vi "3458A Digitizing Process.vi"(8 "error in":errorcluster, 11 "session in":variant) -> (0 "error out":errorcluster, 3 "aux data out":variant)   [LabVIEW 2018, in "3458A Virtual Digitizer.lvlib"]
doc: "3458A digitizing lib: Main digitizing process. The VI is assynchronously executed once for each channel (all in parallel). It is started by calling 'Initiate Digitizing Process'. It then samples and sends the digitized data via queues to main process where the data are collected using 'Fetch Digitized Data'. Configuration of the execution is stored in 'session in' variable, execution control details are in 'session in->proc setup' cluster. Each instance of this VI has ID starting from 0 which identifies to which channel it belongs to."
uses:
  3458A Virtual Digitizer.lvlib
  3458A Digitizer Session.ctl
  3458A Virtual Channel Config.ctl
  Counter/Counter Session.ctl
  Counter/Counter Type.ctl
  AWG/AWG Session.ctl
  AWG/AWG Type.ctl
  3458A Sync Mode.ctl
  3458A Idn Mode.ctl
  3458A Digitizing Low Levels/Configure/Sampling Mode.ctl
  3458A Digitizing Process Options.ctl
  3458A Data Packet.ctl
  3458A Aux Record Data.ctl
  3458A Digitizing Low Levels/Configure/Level Setup.ctl
  3458A Digitizing Low Levels/Configure/First Sample Trigger.ctl
  3458A Aperture Selection Mode.ctl
  <vilib>/Utility/error.llb/Error Cluster From Error Code.vi
  <vilib>/ErrorRing/Error Ring.xnode
  Counter/Counter.lvlib
  AWG/AWG.lvlib
  3458A Digitizing Low Levels/3458A Digitizing Low Levels.lvlib
  3458A Basic Driver/3458A Basic Driver.lvlib
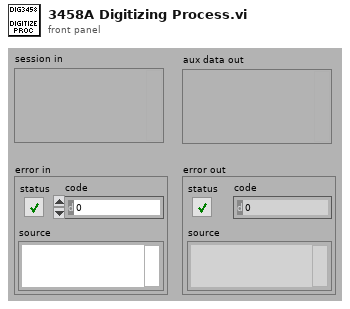
[diagram p1: front panel]
types:
  T1 = typedef "3458A Virtual Digitizer.lvlib/3458A Digitizing Low Levels.lvlib/First Sample Trigger.ctl" = enum16{"AUTO", "EXT", "SYN", "SGL", "HOLD", "LEVEL"}
  T2 = typedef "3458A Virtual Digitizer.lvlib/3458A Data Packet.ctl" = cluster{"data":i32[][], "offset [smpl]":i32, "count [smpl]":i32, "all done?":bool, "sampling?":bool, "queue buffer [%]":dbl, "valid?":bool}
  T3 = typedef "3458A Virtual Digitizer.lvlib/3458A Digitizer Session.ctl" = cluster{"channels":T4[], "sync unit":T5, "awg unit":T7, "sync mode":T9, "streaming mode":bool, "idn mode":T10, "sampling mode":T11, "Ts [s]":dbl, "sample memory [B]":i32, "proc setup":T12, "sample size [B]":i32, "sample count":i32, "aux data":T14, "ranges [V]":dbl[], "aperture [s]":dbl, "LEVEL trigger":T15, "trigger mode":T1, "measure temp.?":bool, "disp mesages":string[], "shared bus?":bool, "disable display?":bool, "aper mode":T16, "aper rules":dbl[][]}
  T4 = typedef "3458A Virtual Digitizer.lvlib/3458A Virtual Channel Config.ctl" = cluster{"VISA":refnum<visa-resource-name>, "Range [Vpk]":dbl, "btn clr":bool, "btn up":bool, "btn down":bool}
  T5 = typedef "Counter.lvlib/Counter Session.ctl" = cluster{"VISA":refnum<visa-resource-name>, "type":T6}
  T6 = typedef "Counter.lvlib/Counter Type.ctl" = enum16{"Picotest U6200A", "dummy"}
  T7 = typedef "AWG.lvlib/AWG Session.ctl" = cluster{"type":T8, "VISA":refnum<visa-resource-name>, "enable 10MHz ref":bool}
  T8 = typedef "AWG.lvlib/AWG Type.ctl" = enum16{"Agilent 331xxA to 332xxA", "Agilent 335xxA to 336xxA", "Tektronix AFG3101C", "dummy"}
  T9 = typedef "3458A Virtual Digitizer.lvlib/3458A Sync Mode.ctl" = enum16{"MASTER-SLAVE, MASTER clocked by TIMER", "MASTER-SLAVE, MASTER clocked by AWG", "ALL clocked by AWG", "MASTER-SLAVE, ALL clocked by TIMER", "ALL clocked by AWG with DFLL"}
  T10 = typedef "3458A Virtual Digitizer.lvlib/3458A Idn Mode.ctl" = enum16{"Auto", "Sequential (chn A, chn B, ...)", "From calibration string"}
  T11 = typedef "3458A Virtual Digitizer.lvlib/3458A Digitizing Low Levels.lvlib/Sampling Mode.ctl" = enum16{"DCV", "DSDC", "DSAC"}
  T12 = typedef "3458A Virtual Digitizer.lvlib/3458A Digitizing Process Options.ctl" = cluster{"channel id":i32, "packet size [smpl]":i32, "current timeout [s]":dbl, "blk2blk timeout [s]":dbl, "event time":timestamp, "stop notifier":refnum<notifier>, "data queues":refnum<queue>[], "proc refs":refnum<vi>[], "bus semaphore":T13}
  T13 = typedef "Semaphore RefNum" = refnum<k1>
  T14 = typedef "3458A Virtual Digitizer.lvlib/3458A Aux Record Data.ctl" = cluster{"channel id":i32, "valid?":bool[], "gain [V]":dbl[], "timestamp [s]":dbl[], "Ts [s]":dbl, "abs timestamp":timestamp, "t [deg C]":dbl[]}
  T15 = typedef "3458A Virtual Digitizer.lvlib/3458A Digitizing Low Levels.lvlib/Level Setup.ctl" = cluster{"edge":enum16{"POS", "NEG"}, "level [V]":dbl, "coupling":enum16{"DC", "AC"}}
  T16 = typedef "3458A Virtual Digitizer.lvlib/3458A Aperture Selection Mode.ctl" = enum16{"Manual", "Maximum", "Table"}
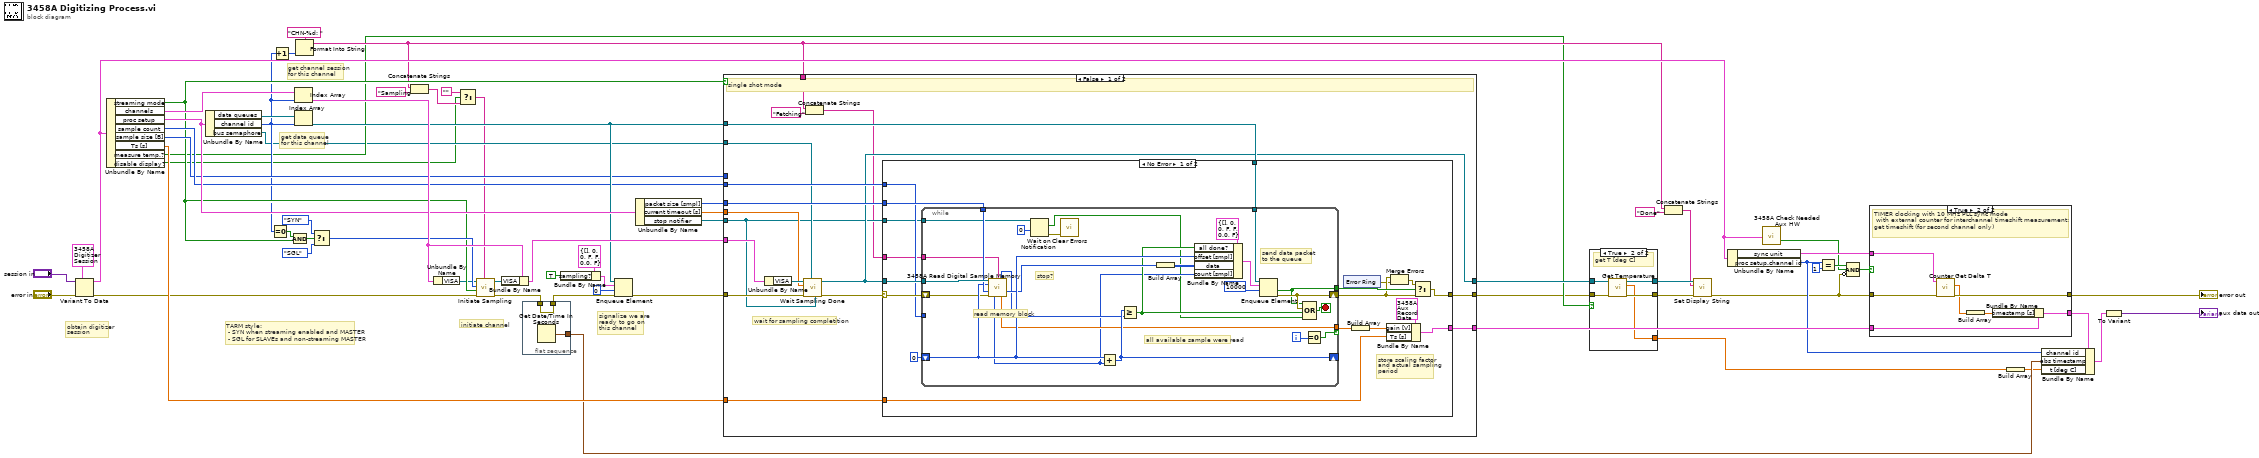
[diagram p0: block diagram]
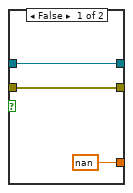
[diagram p2: hidden frame]
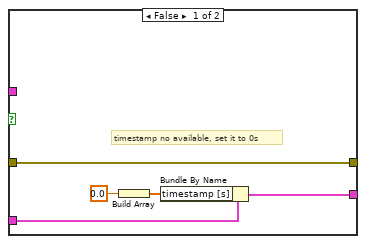
[diagram p3: hidden frame]
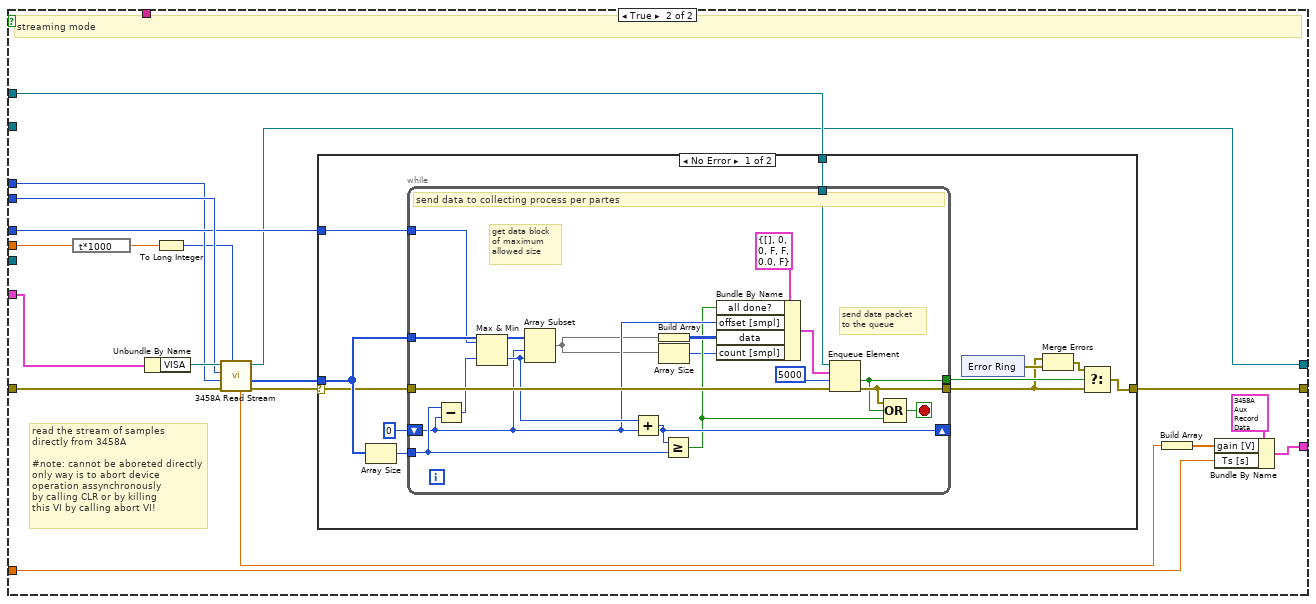
[diagram p5: hidden frame]
diagram:
  # "TARM style:\n - SYN when streaming enabled and MASTER\n - SGL for SLAVEs and non-streaming MASTER"
  # "get channel session\nfor this channel"
  # "get data queue\nfor this channel"
  # "signalize we are\nready to go on \nthis channel"
  # "initiate channel"
  # "obtain digitizer\nsession"
  n1 = Variant To Data(error in="error in", type=T3 {"channels"=[], "sync unit"={"VISA"="", "type"=enum."Picotest U6200A"}, "awg unit"={"type"=enum."Agilent 331xxA to 332xxA", "VISA"="", "enable 10MHz ref"=FALSE}, "sync mode"=enum."MASTER-SLAVE, MASTER clocked by TIMER", "streaming mode"=FALSE, "idn mode"=enum."Auto", "sampling mode"=enum."DCV", "Ts [s]"=0.0, "sample memory [B]"=0, "proc setup"={"channel id"=0, "packet size [smpl]"=0, "current timeout [s]"=0.0, "blk2blk timeout [s]"=0.0, "event time"=timestamp(0 s since 1904-01-01), "stop notifier"=refnum, "data queues"=[], "proc refs"=[], "bus semaphore"=refnum}, "sample size [B]"=0, "sample count"=0, "aux data"={"channel id"=0, "valid?"=[], "gain [V]"=[], "timestamp [s]"=[], "Ts [s]"=0.0, "abs timestamp"=timestamp(0 s since 1904-01-01), "t [deg C]"=[]}, "ranges [V]"=[], "aperture [s]"=0.0, "LEVEL trigger"={"edge"=enum."POS", "level [V]"=0.0, "coupling"=enum."DC"}, "trigger mode"=enum."AUTO", "measure temp.?"=FALSE, "disp mesages"=[], "shared bus?"=FALSE, "disable display?"=FALSE, "aper mode"=enum."Manual", "aper rules"=[]} ("digitizer session"), Variant="session in") -> (data=w42:T3, error out=w20:errorcluster)
  n2 = Unbundle By Name(w42) -> ("streaming mode"=w25:bool, "channels"=w62:T4[], "proc setup"=w54:T12, "sample count"=w49:i32, "sample size [B]"=w34:i32, "Ts [s]"=w29:dbl, "measure temp.?"=w9:bool, "disable display?"=w2:bool)
  n3 = Unbundle By Name(w54) -> ("data queues"=w61:refnum<queue>[], "channel id"=w16:i32, "bus semaphore"=w7:T13)
  n4 = Equal To 0?(x=w16) -> (x = 0?=w32:bool)
  n5 = Increment(x=w16) -> (x+1=w15:i32)
  n6 = Compound Arithmetic op=AND(w32, w25) -> (w33:bool)
  n7 = Index Array(array=w62, index=w16) -> (element=w60:T4)
  n8 = Index Array(array=w61, index=w16) -> (element=w50:refnum<queue>)
  n9 = Format Into String(format string="CHN-%d: ", w15) -> (resulting string=w10:string)  [unwired: 2 in, 1 out]
  n10 = Select(t=First_Sample_Trigger."SYN" ("ARM mode (SGL)"), s=w33, f=First_Sample_Trigger."SGL" ("ARM mode (SGL)")) -> (s? t:f=w26:T1)
  n11 = Concatenate Strings(w10, "Sampling" ("string")) -> (w3:string)
  n12 = Unbundle By Name(w60) -> ("VISA"=w19:refnum<visa-resource-name>)
  n13 = Select(t="", s=w2, f=w3) -> (s? t:f=w4:string)
  n14 = call "Initiate Sampling.vi"("display string (none)"=w4, "error in"=w20, "stream mode (False)"=w25, "ARM mode (SGL)"=w26, "VISA resource in"=w19) -> ("error out"=w28:errorcluster, "VISA resource out"=w35:refnum<visa-resource-name>)  [unwired: 5 in]
  n15 = Bundle By Name(cluster=w60, "VISA"=w35) -> (w55:T4)
  n16 = flat-sequence {
    tunnel: w28 -> [w66]
    tunnel: [w66] -> w27
    tunnel: [w65] -> w23
    frame #0 {
      n17 = Get Date/Time In Seconds() -> (seconds since 1Jan1904=w65:timestamp)
    }
  }
  n18 = Bundle By Name(cluster=T2 {"data"=[], "offset [smpl]"=0, "count [smpl]"=0, "all done?"=FALSE, "sampling?"=FALSE, "queue buffer [%]"=0.0, "valid?"=FALSE} ("niScope packet"), "sampling?"=TRUE) -> (w57:T2)
  n19 = Enqueue Element(queue=w50, element=w57, timeout in ms (-1)=0, error in (no error)=w27) -> (error out=w36:errorcluster)  [unwired: 2 out]
  n20 = Unbundle By Name(w54) -> ("packet size [smpl]"=w51:i32, "current timeout [s]"=w53:dbl, "stop notifier"=w52:refnum<notifier>)
  n21 = case shown="False" w25 {
    tunnel: w36 -> [w75 w151]
    tunnel: w55 -> [w81 w150]
    tunnel: w53 -> [w82 w142]
    tunnel: w52 -> [w68 _]
    tunnel: w51 -> [w80 w139]
    tunnel: w50 -> [w79 w147]
    tunnel: w49 -> [w78 w148]
    tunnel: [w77 w138] -> w6
    tunnel: [w76 w145] -> w43
    tunnel: w34 -> [_ w137]
    tunnel: w29 -> [w74 w133]
    tunnel: [w70 w134] -> w24
    tunnel: w10 -> [w72 _]
    tunnel: w7 -> [w69 _]
    frame False {
      # "wait for sampling completition"
      # "single shot mode"
      n22 = Unbundle By Name(w81) -> ("VISA"=w83:refnum<visa-resource-name>)
      n23 = call "Wait Sampling Done.vi"("stop notifier ref (none)"=w68, "semaphore"=w69, "error in"=w75, "timeout [s] (5s)"=w82, "VISA resource in"=w83) -> ("error out"=w71:errorcluster, "VISA resource out"=w70:refnum<visa-resource-name>)  [unwired: 5 in]
      n24 = Concatenate Strings(w72, "Fetching" ("string")) -> (w67:string)
      n25 = case shown="No Error" w71 {
        selector: w71 -> [w100 w132]
        tunnel: w70 -> [w101 _]
        tunnel: w80 -> [w98 _]
        tunnel: w79 -> [w97 _]
        tunnel: w78 -> [w96 _]
        tunnel: [w90 w132] -> w77
        tunnel: [w93 _] -> w76
        tunnel: w74 -> [w86 _]
        tunnel: w67 -> [w85 _]
        tunnel: w68 -> [w84 _]
        frame No Error {
          # "store scaling factor\nand actual sampling\nperiod"
          n26 = while {
            tunnel: w101 -> [w128]
            shift-right: [w119] -> w88
            shift-left: w100 -> [w111]
            shift-right: [w123] -> _
            shift-left: 0 -> [w125]
            tunnel: w98 -> [w127]
            tunnel: w97 -> [w126]
            tunnel: w96 -> [_]
            tunnel: [w122] -> w94 if=w120
            tunnel: [w115] -> w91
            tunnel: w85 -> [w112]
            tunnel: w84 -> [w110]
            i -> [w121]
            stop <- w117 stop-if-true
            # "stop?"
            # "all available sample were read"
            # "read memory block"
            # "send data packet\nto the queue"
            n27 = call "3458A Read Digital Sample Memory.vi"("VISA session"=w128, "display string (none)"=w112, "First Read in Memory Location (0)"=w125, "max read [smpl]"=w127, "error in (no error)"=w111) -> ("total samples in memory?"=w114:i32, "waveform data int32"=w124:i32[], "read samples"=w113:i32, "scale factor"=w122:dbl)  [unwired: 4 in, 3 out]
            n28 = Wait on Notification(notifier=w110, timeout in ms (-1)=0) -> (notification=w107:bool, error out=w109:errorcluster)  [unwired: 2 in, 2 out]
            n29 = call <vilib>:"Clear Errors.vi"("error in (no error)"=w109) -> ()  [unwired: 5 in, 2 out]
            n30 = Add(x=w125, y=w113) -> (x+y=w123:i32)
            n31 = Greater Or Equal?(x=w123, y=w114) -> (x >= y?=w118:bool)
            n32 = Build Array(w124) -> (w116:i32[][])
            n33 = Bundle By Name(cluster=T2 {"data"=[], "offset [smpl]"=0, "count [smpl]"=0, "all done?"=FALSE, "sampling?"=FALSE, "queue buffer [%]"=0.0, "valid?"=FALSE} ("niScope packet"), "all done?"=w118, "offset [smpl]"=w125, "data"=w116, "count [smpl]"=w113) -> (w130:T2)
            n34 = Enqueue Element(queue=w126, element=w130, timeout in ms (-1)=10000) -> (timed out?=w115:bool, error out=w119:errorcluster)  [unwired: 1 in, 1 out]
            n35 = Compound Arithmetic op=OR(w115, w119, w118, w107) -> (w117:bool)
            n36 = Equal To 0?(x=w121) -> (x = 0?=w120:bool)
          }
          n37 = xnode "Error Ring"() -> ("error out"=w87:errorcluster)
          n38 = Build Array(w94) -> (w92:dbl[])
          n39 = Bundle By Name(cluster=T14 {"channel id"=0, "valid?"=[], "gain [V]"=[], "timestamp [s]"=[], "Ts [s]"=0.0, "abs timestamp"=timestamp(0 s since 1904-01-01), "t [deg C]"=[]} ("aux data"), "gain [V]"=w92, "Ts [s]"=w86) -> (w93:T14)
          n40 = Merge Errors(w88, w87) -> (w89:errorcluster)
          n41 = Select(t=w89, s=w91, f=w88) -> (s? t:f=w90:errorcluster)
        }
        frame Error {
          # "timeout occured, do nothing"
        }
      }
    }
    frame True {
      # "read the stream of samples\ndirectly from 3458A\n\n#note: cannot be aboreted directly\nonly way is to abort device\noperation assynchronously\nby calling CLR or by killing\nthis VI by calling abort VI!"
      # "streaming mode"
      n42 = expression code="t*1000"(w142) -> (w141:dbl)
      n43 = Unbundle By Name(w150) -> ("VISA"=w149:refnum<visa-resource-name>)
      n44 = To Long Integer(number=w141) -> (32bit integer=w135:i32)
      n45 = call "3458A Read Stream.vi"("read timeout [ms] (30000s)"=w135, "error in (no error)"=w151, "sample size [B]"=w137, "samples count"=w148, "VISA session"=w149) -> ("error out"=w136:errorcluster, "waveform data int32"=w140:i32[], "dup VISA session"=w134:refnum<visa-resource-name>, "scale factor"=w144:dbl)  [unwired: 1 in, 2 out]
      n46 = case shown="No Error" w136 {
        selector: w136 -> [w154 w187]
        tunnel: w147 -> [w162 _]
        tunnel: w140 -> [w160 _]
        tunnel: w139 -> [w159 _]
        tunnel: [w155 w187] -> w138
        frame No Error {
          n47 = Array Size(array=w160) -> (size(s)=w153:i32)
          n48 = while {
            tunnel: w154 -> [w183]
            tunnel: [w178] -> w152
            tunnel: w162 -> [w182]
            tunnel: w160 -> [w180]
            shift-right: [w179] -> _
            shift-left: 0 -> [w171]
            tunnel: w159 -> [w174]
            tunnel: w153 -> [w175]
            tunnel: [w176] -> w156
            stop <- w177 stop-if-true
            # "get data block\nof maximum\nallowed size"
            # "send data packet\nto the queue"
            # "send data to collecting process per partes"
            n49 = Subtract(x=w175, y=w171) -> (x-y=w173:i32)
            n50 = Max & Min(x=w174, y=w173) -> (min(x,y)=w172:i32)  [unwired: 1 out]
            n51 = Array Subset(array=w180, index=w171, length=w172) -> (w168:i32[])
            n52 = Add(x=w172, y=w171) -> (x+y=w179:i32)
            n53 = Build Array(w168) -> (w181:i32[][])
            n54 = Array Size(array=w168) -> (size(s)=w169:i32)
            n55 = Greater Or Equal?(x=w179, y=w175) -> (x >= y?=w170:bool)
            n56 = Bundle By Name(cluster=T2 {"data"=[], "offset [smpl]"=0, "count [smpl]"=0, "all done?"=FALSE, "sampling?"=FALSE, "queue buffer [%]"=0.0, "valid?"=FALSE} ("niScope packet"), "all done?"=w170, "offset [smpl]"=w171, "data"=w181, "count [smpl]"=w169) -> (w185:T2)
            n57 = Enqueue Element(queue=w182, element=w185, timeout in ms (-1)=5000, error in (no error)=w183) -> (timed out?=w176:bool, error out=w178:errorcluster)  [unwired: 1 out]
            n58 = Compound Arithmetic op=OR(w178, w176, w170) -> (w177:bool)
          }
          n59 = xnode "Error Ring"() -> ("error out"=w157:errorcluster)
          n60 = Merge Errors(w152, w157) -> (w158:errorcluster)
          n61 = Select(t=w158, s=w156, f=w152) -> (s? t:f=w155:errorcluster)
        }
        frame Error {
        }
      }
      n62 = Build Array(w144) -> (w146:dbl[])
      n63 = Bundle By Name(cluster=T14 {"channel id"=0, "valid?"=[], "gain [V]"=[], "timestamp [s]"=[], "Ts [s]"=0.0, "abs timestamp"=timestamp(0 s since 1904-01-01), "t [deg C]"=[]} ("aux data"), "gain [V]"=w146, "Ts [s]"=w133) -> (w145:T14)
    }
  }
  n64 = case shown="True" w9 {
    tunnel: w6 -> [w189 w195]
    tunnel: [w189 w194] -> w18
    tunnel: [w190 w193] -> w17
    tunnel: w24 -> [w190 w192]
    tunnel: [nan w191] -> w22
    frame False {
    }
    frame True {
      # "get T [deg C]"
      n65 = call "Get Temperature.vi"("error in(no error)"=w195, "VISA Resource Name"=w192) -> ("error out"=w194:errorcluster, "temperature [deg C]"=w191:dbl, "VISA resource name out"=w193:refnum<visa-resource-name>)  [unwired: 7 in]
    }
  }
  n66 = Concatenate Strings(w10, "Done" ("string")) -> (w12:string)
  n67 = call "Set Display String.vi"("error in(no error)"=w18, "display string (none)"=w12, "VISA Resource Name"=w17) -> ("error out"=w5:errorcluster)  [unwired: 7 in, 1 out]
  n68 = Unbundle By Name(w42) -> ("sync unit"=w46:T5, "proc setup.channel id"=w37:i32)
  n69 = call "3458A Check Needed Aux HW.vi"("digitizer session"=w42) -> ("uses counter for delta T sync?"=w41:bool)  [unwired: 13 in, 5 out]
  n70 = Equal?(x=w37, y=1) -> (x = y?=w44:bool)
  n71 = Compound Arithmetic op=AND(w44, w41, invert w5) -> (w47:bool)
  n72 = case shown="True" w47 {
    tunnel: w5 -> [w200 w204]
    tunnel: w46 -> [_ w202]
    tunnel: w43 -> [w198 w207]
    tunnel: [w200 w203] -> w8
    tunnel: [w199 w206] -> w38
    frame False {
      # "timestamp no available, set it to 0s"
      n73 = Build Array(0.0 ("time stamp [s]")) -> (w197:dbl[])
      n74 = Bundle By Name(cluster=w198, "timestamp [s]"=w197) -> (w199:T14)
    }
    frame True {
      # "TIMER clocking with 10 MHz PLL sync mode\n with external counter for interchannel timeshift measurement:\nget timeshift (for second channel only)"
      n75 = call "Counter Get Delta T.vi"("error in"=w204, "counter session in"=w202) -> ("error out"=w203:errorcluster, "delta t [s]"=w201:dbl)  [unwired: 7 in, 1 out]
      n76 = Build Array(w201) -> (w205:dbl[])
      n77 = Bundle By Name(cluster=w207, "timestamp [s]"=w205) -> (w206:T14)
    }
  }
  "error out" <- w8
  n78 = Build Array(w22) -> (w21:dbl[])
  n79 = Bundle By Name(cluster=w38, "channel id"=w37, "abs timestamp"=w23, "t [deg C]"=w21) -> (w39:T14)
  n80 = To Variant(anything=w39) -> (Variant=→"aux data out":variant)
